vi "main.vi"() -> ()   [LabVIEW 2015]
uses:
  typedefs/PLC Cluster.ctl
  <vilib>/DATA AHEAD/SP7/typedefs/PLC Type.ctl
  <vilib>/DATA AHEAD/SP7/functions/read/read int array.vi
  <vilib>/DATA AHEAD/SP7/SP7.lvlib
panel:
  out "Connected?":bool
  in  "PLC":T1={"IP address "="", "PLC Type"=enum."S7 300/400"}
  in  "Connect Button":bool
  in  "Stop Button":bool
  in  "Start Button":bool
  out "Waveform Chart":dbl[](graph)
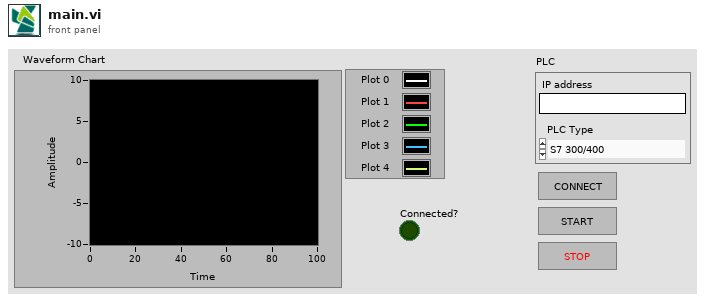
[diagram p1: front panel]
types:
  T1 = typedef "PLC Cluster.ctl" = cluster{"IP address ":string, "PLC Type":T2}
  T2 = typedef "SP7.lvlib/PLC Type.ctl" = enum16{"S7 200", "S7 300/400", "S7 1200", "S7 1500"}
  T3 = typedef "SP7.lvlib/S7 Connection.ctl" = cluster{"TCP Connection Ref":refnum<k5>, "IP address":string, "timeout ms":i32, "Connected?":bool, "PLC Type":T2}
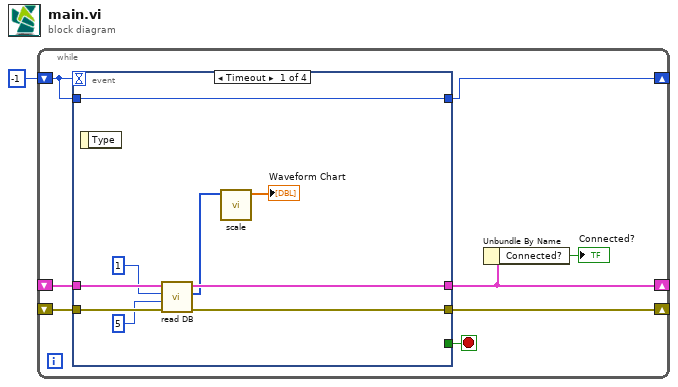
[diagram p0: block diagram]
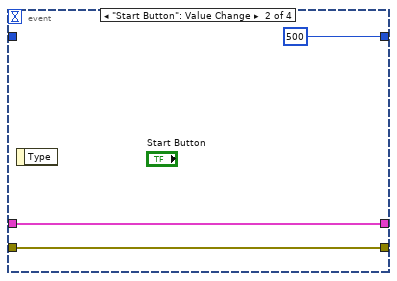
[diagram p2: hidden frame]
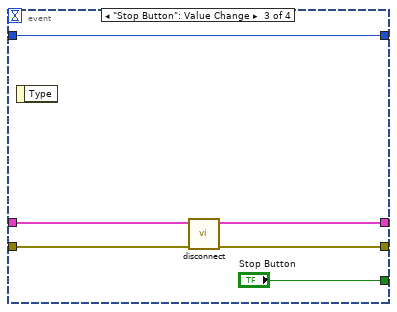
[diagram p3: hidden frame]
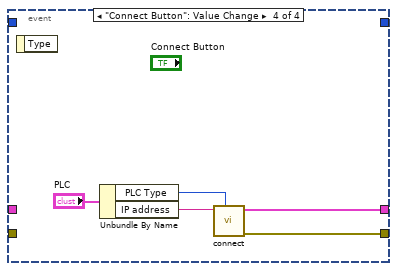
[diagram p4: hidden frame]
diagram:
  n1 = while {
    shift-right: [w8] -> _
    shift-left: -1 -> [w9]
    shift-right: [w3] -> _
    shift-left: _ -> [w6]
    shift-right: [w5] -> _
    shift-left: _ -> [w4]
    stop <- w7 stop-if-true
    n2 = event shown="[0] Timeout" {
      selector: _ -> [_ _ _ _]
      dyn-events: _ -> [_ _ _ _]
      timeout: w9 -> [_ _ _ _]
      tunnel: [w18 500 w26 _] -> w8
      tunnel: w9 -> [w18 _ w26 _]
      tunnel: [_ _ "Stop Button" _] -> w7
      tunnel: [w16 w21 w22 w32] -> w3
      tunnel: w6 -> [w17 w21 w23 _]
      tunnel: [w15 w20 w24 w31] -> w5
      tunnel: w4 -> [w14 w20 w25 _]
      event Timeout {
        n3 = event-data() -> ()  [unwired: 1 in, 1 out]
        n4 = call-poly <vilib>:"read DB.vi"("error in (no error)"=w14, "items #"=u16 5, "Data Block #"=u16 1, "S7 Connection in"=w17) -> ("error out"=w15:errorcluster, "Int result array"=w11:i16[], "S7 Connection out"=w16:T3)  [unwired: 5 in]
        n5 = call "scale.vi"("Int result array"=w11) -> ("Scaled result"=→"Waveform Chart":dbl[])  [unwired: 10 in]
      }
      event "Start Button": Value Change {
        n6 = event-data() -> ()  [unwired: 1 in, 1 out]
      }
      event "Stop Button": Value Change {
        n7 = event-data() -> ()  [unwired: 1 in, 1 out]
        n8 = call <vilib>:"disconnect.vi"("error in (no error)"=w25, "S7 Connection in"=w23) -> ("error out"=w24:errorcluster, "S7 Connection out"=w22:T3)  [unwired: 8 in]
      }
      event "Connect Button": Value Change {
        n9 = event-data() -> ()  [unwired: 1 in, 1 out]
        n10 = Unbundle By Name("PLC") -> ("PLC Type"=w28:T2, "IP address"=w29:string)
        n11 = call <vilib>:"connect.vi"("PLC Type"=w28, "IP address"=w29) -> ("error out"=w31:errorcluster, "S7 Connection out"=w32:T3)  [unwired: 8 in]
      }
    }
    n12 = Unbundle By Name(w3) -> ("Connected?"=→"Connected?":bool)
  }
